vi "Get_Cap.vi"(8 "error in (no error)":errorcluster, 11 "VISA Refnum in":refnum<visa-resource-name>) -> (0 "error out":errorcluster, 1 "String":string, 2 "Numeric":dbl, 3 "VISA Refnum out":refnum<visa-resource-name>)   [LabVIEW 2017]
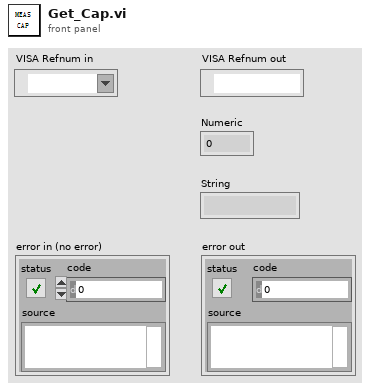
[diagram p1: front panel]
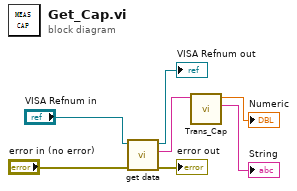
[diagram p0: block diagram]
diagram:
  n1 = call "get data.vi"("错误输入（无错误）"="error in (no error)", "VISA GPIB Resource"="VISA Refnum in") -> ("错误输出"=→"error out":errorcluster, "Read Buffer"=w5:string, "VISA资源名称输出"=→"VISA Refnum out":refnum<visa-resource-name>)  [unwired: 6 in, 1 out]
  n2 = call "Trans_Cap.vi"("Read Buffer"=w5) -> ("String"=→"String":string, "Numeric"=→"Numeric":dbl)  [unwired: 9 in]
